vi "Periodic Tasks.vi"(8 "error in":errorcluster) -> ()   [LabVIEW 2013]
doc: "This VI runs in parallel to other tasks. It can contain as many user-defined periodic loops as you need. These can carry out PID or other sorts of timed response."
uses:
  <vilib>/Rock Robotics/WPI/CAN/Jaguar/SubVIs/WPI_CANJaguar_StatusChannelSelect.ctl
  <vilib>/Rock Robotics/WPI/CAN/Jaguar/SubVIs/WPI_CANJaguar_StatusSelect.ctl
  <vilib>/Rock Robotics/WPI/Joystick/WPI_JoystickGetSetRefNum.vi
  Robot Global Data.vi
  <vilib>/Rock Robotics/WPI/Solenoid/Deprecated/WPI_SolenoidSetBool.vi
  <vilib>/functionblocks/FB Core/FB Core.xnode
  <vilib>/functionblocks/Counter/Timer Off Delay/Timer Off Delay.vi
  <vilib>/functionblocks/NI_FunctionBlock Libraries.lvlib
  <vilib>/functionblocks/Edge Detection/One Shot Falling With Input/One Shot Falling With Input.vi
  <vilib>/functionblocks/Edge Detection/One Shot Rising with Input/One Shot Rising with Input.vi
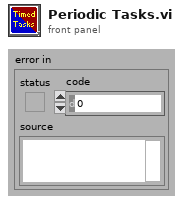
[diagram p1: front panel]
types:
  T1 = typedef "WPI_CompressorDevRef.ctl" = cluster{"DevStatus":errorcluster, "DigitalInputDevRef":T2, "RelayDevRef":T5}
  T2 = typedef "WPI_DigitalInputDevRef.ctl" = cluster{"DevStatus":errorcluster, "DIO Channel":T3, "Digital Module":T4}
  T3 = typedef "FPGA_DIOChannel.ctl" = enum8{"DIO 1", "DIO 2", "DIO 3", "DIO 4", "DIO 5", "DIO 6", "DIO 7", "DIO 8", "DIO 9", "DIO 10", "DIO 11", "DIO 12", "DIO 13", "DIO 14", "Invalid"}
  T4 = typedef "FPGA_TypedefDigitalModule.ctl" = enum16{"Digital Module 1", "Digital Module 2"}
  T5 = typedef "WPI_RelayDevRef.ctl" = cluster{"DevStatus":errorcluster, "Relay Channel":T6, "Digital Module":T4, "Relay Direction":T7}
  T6 = typedef "FPGA_DIORelayChannel.ctl" = enum8{"Relay 1", "Relay 2", "Relay 3", "Relay 4", "Relay 5", "Relay 6", "Relay 7", "Relay 8", "Invalid"}
  T7 = typedef "WPI_RelayDirection.ctl" = enum16{"Both directions", "Forward only", "Reverse only"}
  T8 = typedef "WPI_JoystickDevRef.ctl" = cluster{"Device":T9}
  T9 = typedef "WPI_JoystickDeviceEnum.ctl" = enum16{"USB 1", "USB 2", "USB 3", "USB 4", "Kinect 1", "Kinect 2"}
  T10 = typedef "WPI_CANJaguar_StatusSelect.ctl" = enum16{"Output Percent VBus", "Output Voltage", "Bus Voltage", "Current", "Temperature", "Position", "Speed", "Limit Switches", "Faults", "Fault Counters", "Power Cycle"}
  T11 = typedef "WPI_CANJaguar_StatusChannelSelect.ctl" = enum16{"Periodic Status Channel 1", "Periodic Status Channel 2", "Periodic Status Channel 3", "Periodic Status Channel 4", "On Demand Status"}
  T12 = typedef "WPI_MotorControlDeviceRef.ctl" = cluster{"DeviceStatus":errorcluster, "Type":enum16{"PWM", "CAN"}, "PWM":cluster{"Digital Module":T4, "PWM Channel":T13, "DeadBand":T14}, "CAN":cluster{"Device Number":u8, "Control Mode":T15, "Semaphore":T16, "Max Vout":dbl}, "Invert":bool, "TransformRef":T17, "InvTransformRef":T17}
  T13 = typedef "FPGA_DIOPWMChannel.ctl" = enum8{"PWM 1", "PWM 2", "PWM 3", "PWM 4", "PWM 5", "PWM 6", "PWM 7", "PWM 8", "PWM 9", "PWM 10", "Invalid"}
  T14 = typedef "WPI_PWMDeadband.ctl" = cluster{"Name":string, "maxPositivePwm":i32, "minPositivePwm":i32, "centerPwm":i32, "maxNegativePwm":i32, "minNegativePwm":i32, "angularRange":u16}
  T15 = typedef "WPI_CANJaguar_ControlMode.ctl" = enum8{"Percent VBus", "Current", "Speed", "Position", "Voltage"}
  T16 = typedef "Semaphore RefNum" = refnum<k1>
  T17 = typedef "WPI_PWMTransform_ConPane.ctl" = refnum<vi>
  T18 = typedef "WPI_CANJaguar_Status.ctl" = cluster{"Output Percent VBus":dbl, "Output Voltage":dbl, "Bus Voltage":dbl, "Current":dbl, "Temperature":dbl, "Position":dbl, "Speed":dbl, "Limits":cluster{"Forward Limit":bool, "Reverse Limit":bool, "Forward Soft Limit":bool, "Reverse Soft Limit":bool, "Sticky Forward Limit":bool, "Sticky Reverse Limit":bool, "Sticky Forward Soft Limit":bool, "Sticky Reverse Soft Limit":bool}, "Faults":cluster{"Current Fault":bool, "Temperature Fault":bool, "Bus Voltage Fault":bool, "Gate Driver Fault":bool, "Comm Fault":bool}, "Fault Counters":cluster{"Current Faults":u8, "Temperature Faults":u8, "Bus Voltage Faults":u8, "Gate Driver Faults":u8, "Comm Faults":u8, "CAN Status":u8, "CAN RX Errors":u8, "CAN TX Errors":u8}, "Power Cycle":bool}
  T19 = typedef "WPI_JoystickButtonState.ctl" = cluster{"Button 1":bool, "Button 2":bool, "Button 3":bool, "Button 4":bool, "Button 5":bool, "Button 6":bool, "Button 7":bool, "Button 8":bool, "Button 9":bool, "Button 10":bool, "Button 11":bool, "Button 12":bool}
  T20 = cluster{"axis 1 (x)":dbl, "axis 2 (y)":dbl, "axis 3 (throttle)":dbl, "axis 4":dbl, "axis 5":dbl, "axis 6":dbl}
  T21 = typedef "WPI_SolenoidDevRef.ctl" = cluster{"DevStatus":errorcluster, "Solenoid Module":T22, "Forward Solenoid Channel":T23, "Reverse Solenoid Channel":T23}
  T22 = typedef "FPGA_TypedefSolenoidModule.ctl" = enum16{"Solenoid Module 1", "Solenoid Module 2"}
  T23 = typedef "WPI_SolenoidChannel.ctl" = enum8{"Solenoid 1", "Solenoid 2", "Solenoid 3", "Solenoid 4", "Solenoid 5", "Solenoid 6", "Solenoid 7", "Solenoid 8", "Invalid"}
  T24 = typedef "WPI_DriverStationRobotMode2.ctl" = enum16{"Autonomous Disabled", "Autonomous Enabled", "Teleop Disabled", "Teleop Enabled", "Timeout", "Finish", "Test Disabled", "Test Enabled"}
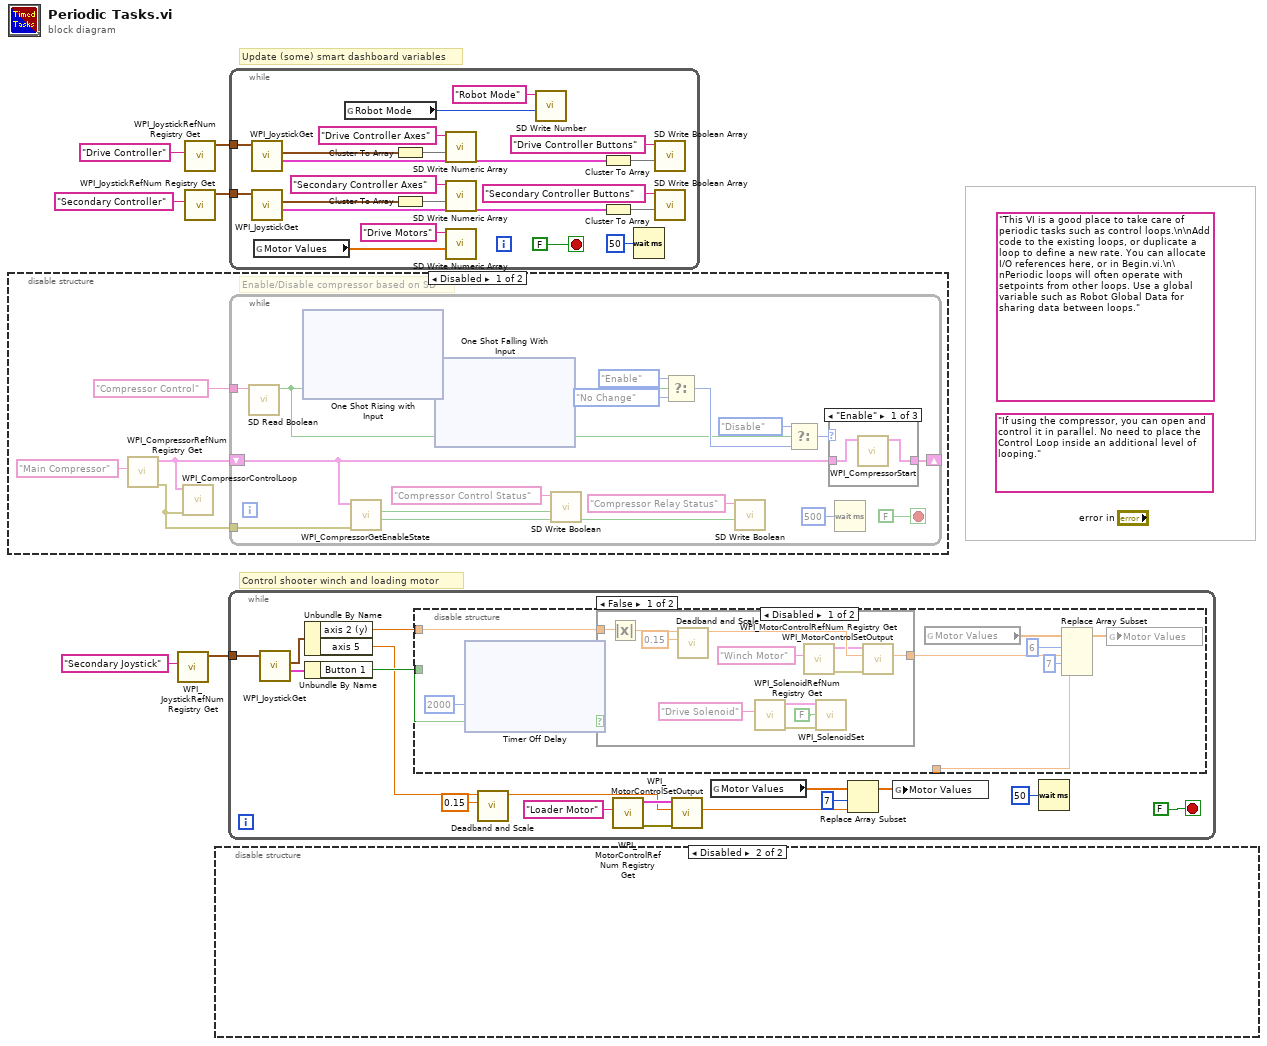
[diagram p0: block diagram]
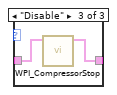
[diagram p3: hidden frame]
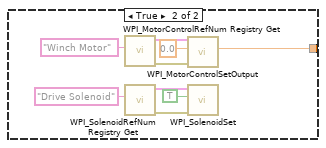
[diagram p5: hidden frame]
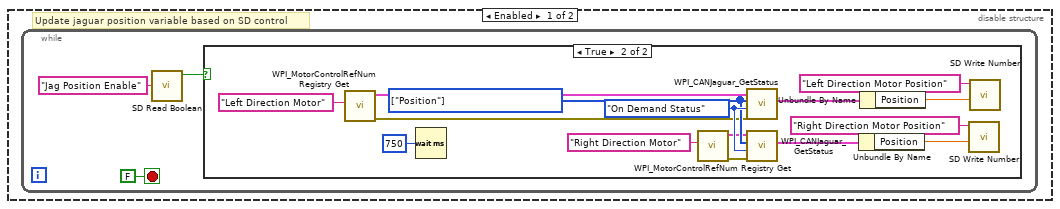
[diagram p7: hidden frame]
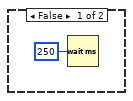
[diagram p8: hidden frame]
diagram:
  (unwired) "If using the compressor, you can open and control it in parallel. No need to place the Control Loop inside an additional level of looping."
  (unwired) "This VI is a good place to take care of periodic tasks such as control loops.\n\nAdd code to the existing loops, or duplicate a loop to define a new rate. You can allocate I/O references here, or in Begin.vi.\n\nPeriodic loops will often operate with setpoints from other loops. Use a global variable such as Robot Global Data for sharing data between loops."
  # "Update (some) smart dashboard variables"
  # "Control shooter winch and loading motor"
  n1 = disable-structure shown="Disabled" {
    frame Disabled {
      # "Enable/Disable compressor based on SD"
      n2 = call <vilib>:"WPI_CompressorRefNum Registry Get.vi"("refnum name"="Main Compressor") -> ("error out"=w7:errorcluster, "CompressorDevRef"=w9:T1)  [unwired: 9 in]
      n3 = call <vilib>:"WPI_CompressorControlLoop.vi"("error in (no error)"=w7, "CompressorDevRef"=w9) -> ()  [unwired: 10 in]
      n4 = while {
        tunnel: "Compressor Control" ("refnum name") -> [w19]
        shift-right: [w15] -> _
        shift-left: w9 -> [w20]
        tunnel: w7 -> [w14]
        stop <- FALSE stop-if-true
        n5 = call <vilib>:"SD Read Boolean.vi"("Name"=w19) -> ("Boolean"=w12:bool)  [unwired: 8 in, 2 out]
        n6 = xnode "One Shot Rising with Input"("input"=w12) -> ("output"=w11:bool)  [unwired: 1 in, 1 out]
        n7 = call <vilib>:"WPI_CompressorGetEnableState.vi"("error in (no error)"=w14, "CompressorDevRef"=w20) -> ("Compressor Running"=w18:bool, "Enabled"=w26:bool)  [unwired: 6 in, 2 out]
        n8 = xnode "One Shot Falling With Input"("input"=w12) -> ("output"=w13:bool)  [unwired: 1 in, 1 out]
        n9 = call <vilib>:"SD Write Boolean.vi"("Boolean"=w26, "Name"="Compressor Control Status") -> ()  [unwired: 8 in, 2 out]
        n10 = Select(t=enum16{"Enable", "No Change", "Disable"}."Enable", s=w11, f=enum16{"Enable", "No Change", "Disable"}."No Change") -> (s? t:f=w24:enum16{"Enable", "No Change", "Disable"})
        n11 = call <vilib>:"SD Write Boolean.vi"("Boolean"=w18, "Name"="Compressor Relay Status") -> ()  [unwired: 8 in, 2 out]
        n12 = Select(t=enum16{"Enable", "No Change", "Disable"}."Disable", s=w13, f=w24) -> (s? t:f=w21:enum16{"Enable", "No Change", "Disable"})
        n13 = case shown="\"Enable\"" w21 {
          tunnel: w20 -> [w106 w107 w109]
          tunnel: [w105 w107 w108] -> w15
          frame "Enable" {
            n14 = call <vilib>:"WPI_CompressorStart.vi"("CompressorDevRef"=w106) -> ("CompressorDevRef"=w105:T1)  [unwired: 9 in, 1 out]
          }
          frame "No Change", Default {
          }
          frame "Disable" {
            n15 = call <vilib>:"WPI_CompressorStop.vi"("CompressorDevRef"=w109) -> ("CompressorDevRef"=w108:T1)  [unwired: 9 in, 1 out]
          }
        }
        n16 = Wait (ms)(milliseconds to wait=u32 500) -> ()  [unwired: 1 out]
      }
    }
    frame Enabled {
    }
  }
  n17 = call <vilib>:"WPI_JoystickRefNum Registry Get.vi"("refnum name"="Secondary Joystick") -> ("JoystickDevRef"=w5:T8)  [unwired: 9 in, 1 out]
  n18 = call <vilib>:"WPI_JoystickRefNum Registry Get.vi"("refnum name"="Drive Controller") -> ("JoystickDevRef"=w4:T8)  [unwired: 9 in, 1 out]
  n19 = call <vilib>:"WPI_JoystickRefNum Registry Get.vi"("refnum name"="Secondary Controller") -> ("JoystickDevRef"=w3:T8)  [unwired: 9 in, 1 out]
  n20 = disable-structure shown="Disabled" {
    frame Enabled {
      # "Update jaguar position variable based on SD control"
      n21 = while {
        stop <- FALSE stop-if-true
        n22 = call <vilib>:"SD Read Boolean.vi"("Name"="Jag Position Enable") -> ("Boolean"=w112:bool)  [unwired: 8 in, 2 out]
        n23 = case shown="True" w112 {
          frame False {
            n24 = Wait (ms)(milliseconds to wait=u32 250) -> ()  [unwired: 1 out]
          }
          frame True {
            w127 = T10[] [enum."Position"] items=["Output Percent VBus", "Output Voltage", "Bus Voltage", "Current", "Temperature", "Position", "Speed", "Limit Switches", "Faults", "Fault Counters", "Power Cycle"] ("Status Select")
            w128 = WPI_CANJaguar_StatusChannelSelect."On Demand Status" ("Status Channel Select")
            n25 = call <vilib>:"WPI_MotorControlRefNum Registry Get.vi"("refnum name"="Left Direction Motor") -> ("error out"=w125:errorcluster, "MotorControlDevRef"=w126:T12)  [unwired: 9 in]
            n26 = Wait (ms)(milliseconds to wait=u32 750) -> ()  [unwired: 1 out]
            n27 = call <vilib>:"WPI_MotorControlRefNum Registry Get.vi"("refnum name"="Right Direction Motor") -> ("error out"=w122:errorcluster, "MotorControlDevRef"=w123:T12)  [unwired: 9 in]
            n28 = call <vilib>:"WPI_CANJaguar_GetStatus.vi"("error in (no error)"=w125, "Status Channel Select"=w128, "Status Select"=w127, "CAN Jaguar Ref"=w126) -> ("Status"=w120:T18)  [unwired: 5 in, 2 out]
            n29 = call <vilib>:"WPI_CANJaguar_GetStatus.vi"("error in (no error)"=w122, "Status Channel Select"=w128, "Status Select"=w127, "CAN Jaguar Ref"=w123) -> ("Status"=w115:T18)  [unwired: 5 in, 2 out]
            n30 = Unbundle By Name(w115) -> ("Position"=w116:dbl)
            n31 = Unbundle By Name(w120) -> ("Position"=w118:dbl)
            n32 = call <vilib>:"SD Write Number.vi"("Numeric"=w116, "Name"="Right Direction Motor Position") -> ()  [unwired: 8 in, 2 out]
            n33 = call <vilib>:"SD Write Number.vi"("Numeric"=w118, "Name"="Left Direction Motor Position") -> ()  [unwired: 8 in, 2 out]
          }
        }
      }
    }
    frame Disabled {
    }
  }
  n34 = while {
    tunnel: w5 -> [w144]
    stop <- FALSE stop-if-true
    n35 = call <vilib>:"WPI_JoystickGet.vi"("JoystickDevRef"=w144) -> ("Buttons"=w142:T19, "Axes"=w143:T20)  [unwired: 4 in, 1 out]
    n36 = Unbundle By Name(w143) -> ("axis 2 (y)"=w134:dbl, "axis 5"=w133:dbl)
    n37 = Unbundle By Name(w142) -> ("Button 1"=w136:bool)
    n38 = disable-structure shown="Disabled" {
      disable-tunnel: w134 -> [w155 _]
      disable-tunnel: _ -> [w149 _]
      disable-tunnel: w136 -> [w147 _]
      frame Disabled {
        n39 = xnode "Timer Off Delay"("preset time (ms)"=2000, "input"=w147) -> ("output"=w146:bool)  [unwired: 1 in, 2 out]
        n40 = case shown="False" w146 {
          tunnel: w155 -> [w205 _]
          tunnel: [w200 w210] -> w152
          frame False {
            n41 = Absolute Value(x=w205) -> (abs(x)=w199:dbl)
            n42 = call "Deadband and Scale.vi"("Dead Zone (abs)"=0.15, "Input"=w199) -> ("Output"=w209:dbl)  [unwired: 9 in]
            n43 = call <vilib>:"WPI_SolenoidRefNum Registry Get.vi"("refnum name"="Drive Solenoid") -> ("error out"=w204:errorcluster, "SolenoidDevRef"=w203:T21)  [unwired: 9 in]
            n44 = call <vilib>:"WPI_MotorControlRefNum Registry Get.vi"("refnum name"="Winch Motor") -> ("error out"=w208:errorcluster, "MotorControlDevRef"=w207:T12)  [unwired: 9 in]
            n45 = call-poly <vilib>:"WPI_SolenoidSet.vi"("error in (no error)"=w204, "Value"=FALSE, "SolenoidDevRef"=w203) -> ()  [unwired: 7 in, 2 out]
            n46 = call <vilib>:"WPI_MotorControlSetOutput.vi"("error in (no error)"=w208, "Output"=w209, "MotorControlDevRef"=w207) -> ("Motor Output"=w200:dbl)  [unwired: 6 in, 2 out]
          }
          frame True {
            n47 = call <vilib>:"WPI_MotorControlRefNum Registry Get.vi"("refnum name"="Winch Motor") -> ("error out"=w214:errorcluster, "MotorControlDevRef"=w213:T12)  [unwired: 9 in]
            n48 = call <vilib>:"WPI_SolenoidRefNum Registry Get.vi"("refnum name"="Drive Solenoid") -> ("error out"=w218:errorcluster, "SolenoidDevRef"=w217:T21)  [unwired: 9 in]
            n49 = call <vilib>:"WPI_MotorControlSetOutput.vi"("error in (no error)"=w214, "Output"=0.0, "MotorControlDevRef"=w213) -> ("Motor Output"=w210:dbl)  [unwired: 6 in, 2 out]
            n50 = call-poly <vilib>:"WPI_SolenoidSet.vi"("error in (no error)"=w218, "Value"=TRUE, "SolenoidDevRef"=w217) -> ()  [unwired: 7 in, 2 out]
          }
        }
        n51 = global read "Robot Global Data.vi" "Motor Values"() -> (w154:dbl[])
        n52 = Replace Array Subset(array=w154, new element #1=w152, index #1=6 ("index"), new element #2=w149, index #2=7 ("index")) -> (w153:dbl[])
        n53 = global write "Robot Global Data.vi" "Motor Values"(w153) -> ()
      }
      frame Enabled {
      }
    }
    n54 = call "Deadband and Scale.vi"("Dead Zone (abs)"=0.15, "Input"=w133) -> ("Output"=w137:dbl)  [unwired: 9 in]
    n55 = call <vilib>:"WPI_MotorControlRefNum Registry Get.vi"("refnum name"="Loader Motor") -> ("error out"=w140:errorcluster, "MotorControlDevRef"=w141:T12)  [unwired: 9 in]
    n56 = call <vilib>:"WPI_MotorControlSetOutput.vi"("error in (no error)"=w140, "Output"=w137, "MotorControlDevRef"=w141) -> ("Motor Output"=w129:dbl)  [unwired: 6 in, 2 out]
    n57 = global read "Robot Global Data.vi" "Motor Values"() -> (w132:dbl[])
    n58 = Replace Array Subset(array=w132, new element=w129, index=7) -> (w131:dbl[])
    n59 = global write "Robot Global Data.vi" "Motor Values"(w131) -> ()
    n60 = Wait (ms)(milliseconds to wait=u32 50) -> ()  [unwired: 1 out]
  }
  n61 = while {
    tunnel: w4 -> [w237]
    tunnel: w3 -> [w236]
    stop <- FALSE stop-if-true
    n62 = call <vilib>:"WPI_JoystickGet.vi"("JoystickDevRef"=w237) -> ("Buttons"=w233:T19, "Axes"=w232:T20)  [unwired: 4 in, 1 out]
    n63 = call <vilib>:"WPI_JoystickGet.vi"("JoystickDevRef"=w236) -> ("Buttons"=w222:T19, "Axes"=w223:T20)  [unwired: 4 in, 1 out]
    n64 = global read "Robot Global Data.vi" "Motor Values"() -> (w235:dbl[])
    n65 = global read "Robot Global Data.vi" "Robot Mode"() -> (w220:T24)
    n66 = Cluster To Array(cluster=w232) -> (array=w230:dbl[])
    n67 = Cluster To Array(cluster=w223) -> (array=w226:dbl[])
    n68 = call <vilib>:"SD Write Numeric Array.vi"("Numeric Array"=w230, "Name"="Drive Controller Axes") -> ()  [unwired: 8 in, 2 out]
    n69 = call <vilib>:"SD Write Numeric Array.vi"("Numeric Array"=w226, "Name"="Secondary Controller Axes") -> ()  [unwired: 8 in, 2 out]
    n70 = call <vilib>:"SD Write Numeric Array.vi"("Numeric Array"=w235, "Name"="Drive Motors") -> ()  [unwired: 8 in, 2 out]
    n71 = call <vilib>:"SD Write Number.vi"("Numeric"=w220, "Name"="Robot Mode") -> ()  [unwired: 8 in, 2 out]
    n72 = Cluster To Array(cluster=w233) -> (array=w231:bool[])
    n73 = Cluster To Array(cluster=w222) -> (array=w227:bool[])
    n74 = Wait (ms)(milliseconds to wait=u32 50) -> ()  [unwired: 1 out]
    n75 = call <vilib>:"SD Write Boolean Array.vi"("Boolean Array"=w231, "Name"="Drive Controller Buttons") -> ()  [unwired: 8 in, 2 out]
    n76 = call <vilib>:"SD Write Boolean Array.vi"("Boolean Array"=w227, "Name"="Secondary Controller Buttons") -> ()  [unwired: 8 in, 2 out]
  }
